vi "SSL_set_bio.vi"(8 "error in (no error)":errorcluster, 10 "BIO":refnum<class "BIO.lvclass">, 11 "SSL in":refnum<class "SSL.lvclass">) -> (0 "error out":errorcluster, 3 "SSL out":refnum<class "SSL.lvclass">)   [LabVIEW 2013, in "SSL_Lib.lvlib" / "SSL.lvclass"]
uses:
  SSL.lvclass
  BIO/BIO.lvclass
  SSL-Lib/SSL-Lib.lvclass/SSL-Lib.ctl
  SSL.lvclass/SSL.ctl
  BIO/BIO.lvclass/BIO.ctl
  BIO/Read Handle.vi
  SSL-Lib/Read SSL Library Path.vi
  Read Handle.vi
  SSL-Lib/SSL-Lib.lvclass
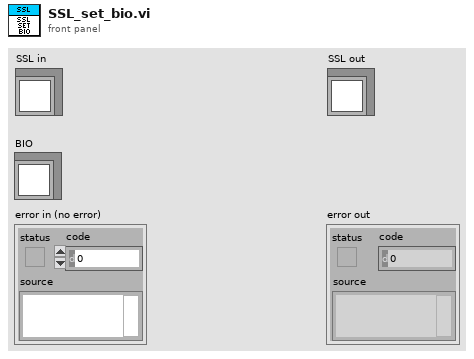
[diagram p1: front panel]
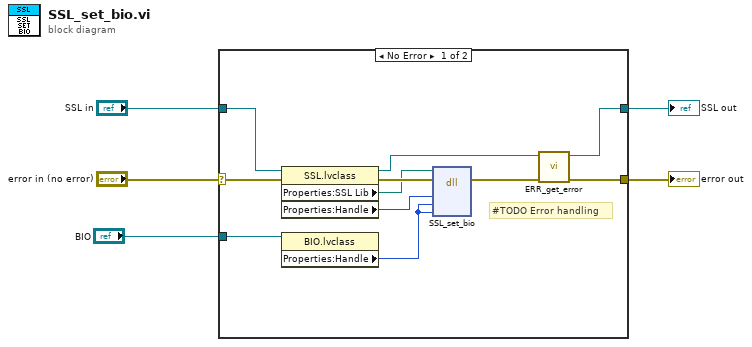
[diagram p0: block diagram]
diagram:
  n1 = case shown="No Error" "error in (no error)" {
    selector: "error in (no error)" -> [w16 w18]
    tunnel: [w11 w18] -> w4
    tunnel: [w9 w17] -> w2
    tunnel: "SSL in" -> [w8 w17]
    tunnel: "BIO" -> [w7 _]
    frame No Error {
      # "#TODO Error handling"
      n2 = property class="SSL.lvclass"(reference=w8, error in=w16) -> (reference out=w10:refnum<class "SSL.lvclass">, error out=w14:errorcluster, "Properties:SSL Lib"=w12:path, "Properties:Handle"=w13:u64)
      n3 = property class="BIO.lvclass"(reference=w7) -> ("Properties:Handle"=w6:u64)  [unwired: 1 in, 2 out]
      n4 = dll-call lib="C:/Program Files (x86)/National Instruments/Shared/nissl/NIssleay32.dll" fn="SSL_set_bio"(path in=w12, error in=w14, "*SSL"=w13, "rbio"=w6, "wbio"=w6) -> (error out=w15:errorcluster)  [unwired: 5 in, 1 out]
      n5 = call "ERR_get_error.vi"("error in (no error)"=w15, "SSL-Lib in"=w10) -> ("error out"=w11:errorcluster, "SSL-Lib out"=w9:refnum<class "SSL.lvclass">)  [unwired: 8 in]
    }
    frame Error {
    }
  }
  "error out" <- w4
  "SSL out" <- w2
